vi "Execute 7z bat.vi"(8 "error in (no error)":errorcluster, 11 "PostBuildSupport in":refnum<class "PostBuildSupport.lvclass">) -> (0 "error out":errorcluster, 3 "PostBuildSupport out":refnum<class "PostBuildSupport.lvclass">)   [LabVIEW 2019, in "PostBuildSupport.lvclass"]
uses:
  PostBuildSupport.lvclass
  PostBuildSupport.lvclass/PostBuildSupport.ctl
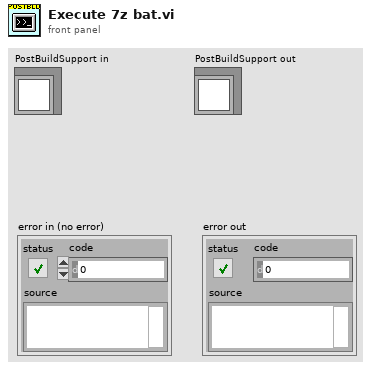
[diagram p1: front panel]
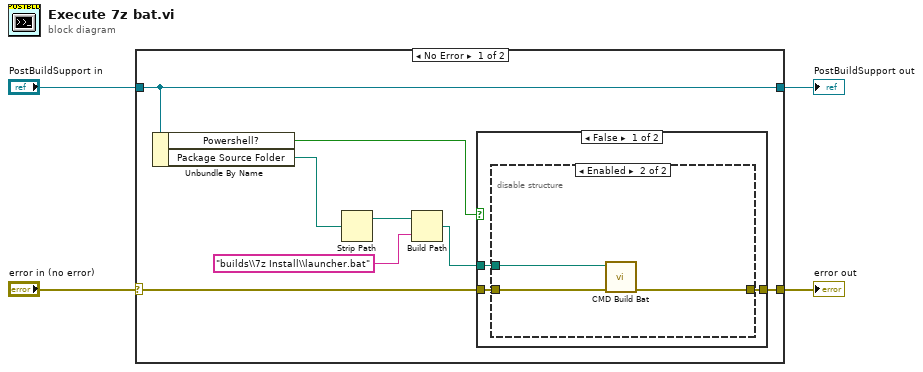
[diagram p0: block diagram]
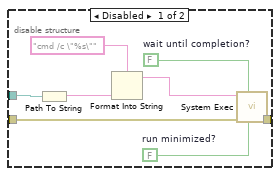
[diagram p2: hidden frame]
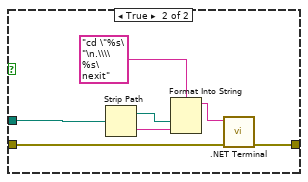
[diagram p3: hidden frame]
diagram:
  n1 = case shown="No Error" "error in (no error)" {
    selector: "error in (no error)" -> [w7 w35]
    tunnel: [w12 w35] -> w1
    tunnel: "PostBuildSupport in" -> [w9 w34]
    tunnel: [w9 w34] -> w3
    frame No Error {
      n2 = Unbundle By Name(w9) -> ("Powershell?"=w6:bool, "Package Source Folder"=w11:path)
      n3 = Strip Path(path=w11) -> (stripped path=w8:path)  [unwired: 1 out]
      n4 = Build Path(base path=w8, name or relative path="builds\\7z Install\\launcher.bat") -> (appended path=w5:path)
      n5 = case shown="False" w6 {
        tunnel: [w15 w31] -> w12
        tunnel: w7 -> [w14 w30]
        tunnel: w5 -> [w13 w29]
        frame False {
          n6 = disable-structure shown="Enabled" {
            disable-tunnel: [w23 w24] -> w15
            disable-tunnel: w14 -> [w22 w25]
            disable-tunnel: w13 -> [w21 w26]
            frame Disabled {
              w17 = FALSE  # run minimized?
              w18 = FALSE  # wait until completion?
              n7 = Path To String(path=w21) -> (string=w20:string)
              n8 = Format Into String(format string="cmd /c \"%s\"", w20) -> (resulting string=w16:string)  [unwired: 2 in, 1 out]
              n9 = call <vilib>:"System Exec.vi"("run minimized? (F)"=w17, "wait until completion? (T)"=w18, "error in (no error)"=w22, "command line"=w16) -> ("error out"=w23:errorcluster)  [unwired: 4 in, 3 out]
            }
            frame Enabled {
              n10 = call "CMD Build Bat.vi"("error in (no error)"=w25, "batch file"=w26) -> ("error out"=w24:errorcluster)  [unwired: 9 in]
            }
          }
        }
        frame True {
          n11 = Strip Path(path=w29) -> (stripped path=w27:path, name=w28:string)
          n12 = Format Into String(format string="cd \"%s\"\n.\\\\%s\nexit", w27, w28) -> (resulting string=w32:string)  [unwired: 2 in, 1 out]
          n13 = call ".NET Terminal.vi"("error in (no error)"=w30, "StdIn"=w32) -> ("error out"=w31:errorcluster)  [unwired: 7 in, 2 out]
        }
      }
    }
    frame Error {
    }
  }
  "error out" <- w1
  "PostBuildSupport out" <- w3
